vi "Timer FGV.vi"(6 "Timer Command":T1, 8 "error in (no error)":errorcluster) -> (0 "error out":errorcluster, 1 "Period":u32)   [LabVIEW 2015]
uses:
  TypeDefs Host/Timer Enum.ctl
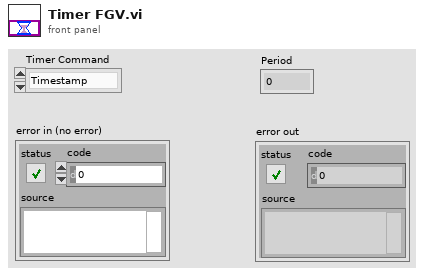
[diagram p1: front panel]
types:
  T1 = typedef "Timer Enum.ctl" = enum16{"Timestamp", "Get Period", "Last Period"}
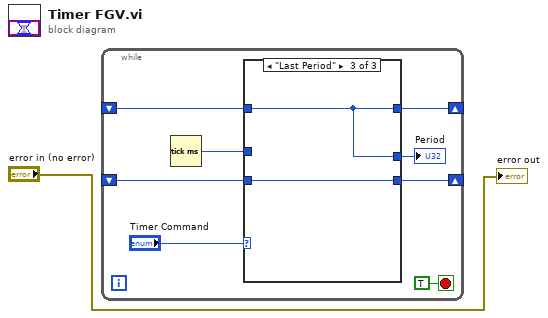
[diagram p0: block diagram]
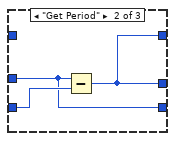
[diagram p3: hidden frame]
diagram:
  n1 = while {
    shift-right: [w8] -> _
    shift-left: _ -> [w7]
    shift-right: [w3] -> _
    shift-left: _ -> [w2]
    stop <- TRUE stop-if-true
    n2 = Tick Count (ms)() -> (millisecond timer value=w5:u32)
    n3 = case shown="\"Last Period\"" "Timer Command" {
      tunnel: [w11 w13 w15] -> w8
      tunnel: w7 -> [_ w14 w15]
      tunnel: w5 -> [w11 w13 _]
      tunnel: [w10 w12 w16] -> w4
      tunnel: [w10 w12 w16] -> w3
      tunnel: w2 -> [w10 _ w16]
      frame "Timestamp", Default {
      }
      frame "Get Period" {
        n4 = Subtract(x=w13, y=w14) -> (x-y=w12:u32)
      }
      frame "Last Period" {
      }
    }
    "Period" <- w4
  }
  "error out" <- "error in (no error)"
